vi "Bai1_6.vi"() -> ()   [LabVIEW 2023]
panel:
  in  "Reset":bool
  in  "Thermometer 8":dbl(slide) scale=0.0..100.0
  out "Led 8":bool
  in  "Thermometer 7":dbl(slide) scale=0.0..100.0
  out "Led 7":bool
  in  "Thermometer 6":dbl(slide) scale=0.0..100.0
  out "Led 6":bool
  in  "Thermometer 5":dbl(slide) scale=0.0..100.0
  out "Led 5":bool
  in  "Thermometer 4":dbl(slide) scale=0.0..100.0
  out "Led 4":bool
  in  "Thermometer 3":dbl(slide) scale=0.0..100.0
  out "Led 3":bool
  in  "Thermometer 2":dbl(slide) scale=0.0..100.0
  out "Led 2":bool
  in  "Thermometer 1":dbl(slide) scale=0.0..100.0
  in  "Stop":bool
  out "Led 1":bool
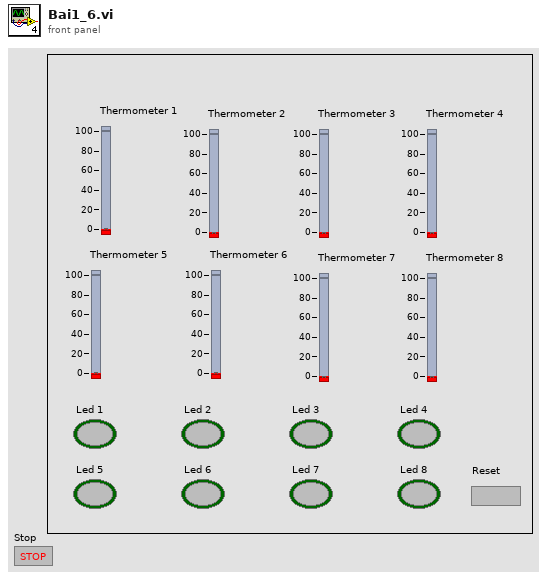
[diagram p1: front panel]
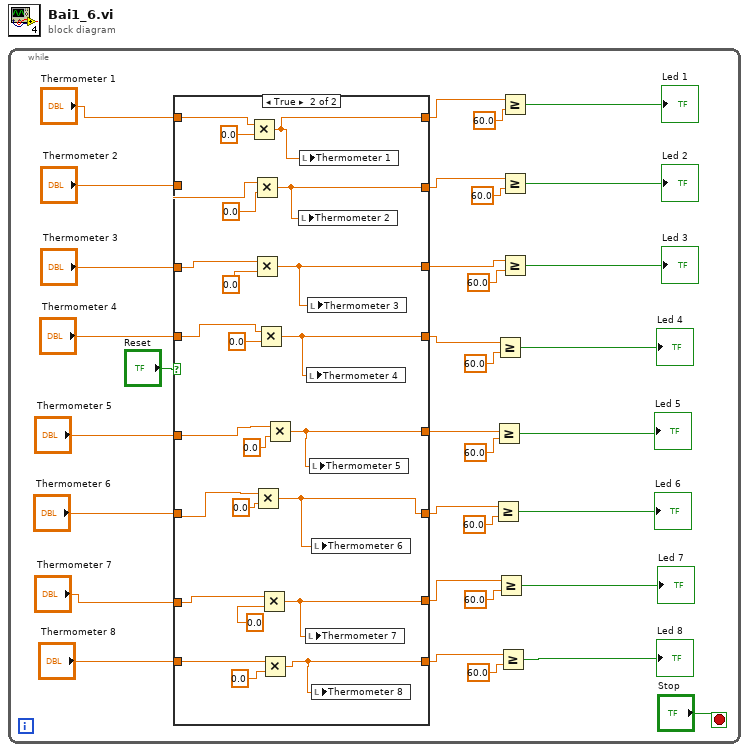
[diagram p0: block diagram]
diagram:
  n1 = while {
    stop <- "Stop" stop-if-true
    n2 = case shown="True" "Reset" {
      tunnel: "Thermometer 1" -> [w42 w59]
      tunnel: "Thermometer 2" -> [w41 w58]
      tunnel: "Thermometer 3" -> [w40 w57]
      tunnel: "Thermometer 4" -> [w39 w54]
      tunnel: "Thermometer 5" -> [w38 w56]
      tunnel: "Thermometer 6" -> [w37 w55]
      tunnel: "Thermometer 7" -> [w36 w53]
      tunnel: "Thermometer 8" -> [w35 w52]
      tunnel: [w42 w50] -> w8
      tunnel: [w41 w49] -> w7
      tunnel: [w40 w48] -> w6
      tunnel: [w39 w47] -> w5
      tunnel: [w38 w46] -> w4
      tunnel: [w37 w45] -> w3
      tunnel: [w36 w44] -> w2
      tunnel: [w35 w43] -> w1
      frame False {
      }
      frame True {
        n3 = Multiply(x=w59, y=0.0) -> (x*y=w50:dbl)
        n4 = Multiply(x=w58, y=0.0) -> (x*y=w49:dbl)
        n5 = Multiply(x=w57, y=0.0) -> (x*y=w48:dbl)
        n6 = Multiply(x=w55, y=0.0) -> (x*y=w45:dbl)
        n7 = Multiply(x=w54, y=0.0) -> (x*y=w47:dbl)
        n8 = Multiply(x=w53, y=0.0) -> (x*y=w44:dbl)
        n9 = Multiply(x=w52, y=0.0) -> (x*y=w43:dbl)
        n10 = Multiply(x=w56, y=0.0) -> (x*y=w46:dbl)
        n11 = local write "Thermometer 2"(w49) -> ()
        n12 = local write "Thermometer 1"(w50) -> ()
        n13 = local write "Thermometer 7"(w44) -> ()
        n14 = local write "Thermometer 4"(w47) -> ()
        n15 = local write "Thermometer 3"(w48) -> ()
        n16 = local write "Thermometer 5"(w46) -> ()
        n17 = local write "Thermometer 6"(w45) -> ()
        n18 = local write "Thermometer 8"(w43) -> ()
      }
    }
    n19 = Greater Or Equal?(x=w3, y=60.0) -> (x >= y?=→"Led 6":bool)
    n20 = Greater Or Equal?(x=w4, y=60.0) -> (x >= y?=→"Led 5":bool)
    n21 = Greater Or Equal?(x=w5, y=60.0) -> (x >= y?=→"Led 4":bool)
    n22 = Greater Or Equal?(x=w2, y=60.0) -> (x >= y?=→"Led 7":bool)
    n23 = Greater Or Equal?(x=w1, y=60.0) -> (x >= y?=→"Led 8":bool)
    n24 = Greater Or Equal?(x=w8, y=60.0) -> (x >= y?=→"Led 1":bool)
    n25 = Greater Or Equal?(x=w7, y=60.0) -> (x >= y?=→"Led 2":bool)
    n26 = Greater Or Equal?(x=w6, y=60.0) -> (x >= y?=→"Led 3":bool)
  }
